vi "Impedance.vi"(7 "Auto Range (F: Off)":bool, 8 "error in (no error)":errorcluster, 9 "Imp Range (Ohm) (0.0)":dbl min=0.0 max=100000000.0 step=1.0 format="%.4f", 10 "Imp Type (0: CPD)":u32(ring) items=["CPD", "CPQ", "CPG", "CPRP", "CSD", "CSQ", "CSRS", "LPQ", "LPD", "LPG", "LPRP", "LSD", "LSQ", "LSRS", "RX", "ZTD", "ZTR", "GB", "YTD", "YTR"], 11 "VISA resource name":refnum<visa-resource-name>) -> (0 "error out":errorcluster, 3 "VISA resource name out":refnum<visa-resource-name>)   [LabVIEW 2015, in "Agilent 428X Series.lvlib"]
doc: "This control sets the measurement range and impedance type. Any value can be used as the setting value. The HP 428XA selects an appropriate measurement range for the setting value.\n\nWarning:\n\nIf this command is received while auto range is ON, the auto range function automatically set to OFF and the range will be held at the range dictated by the received command."
uses:
  Agilent 428X Series.lvlib
panel:
  # "On\nOff"
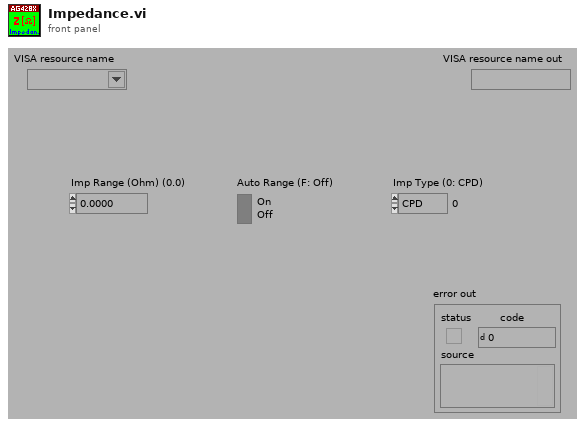
[diagram p1: front panel]
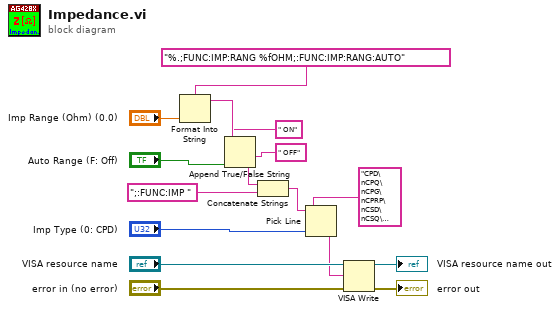
[diagram p0: block diagram]
diagram:
  n1 = Format Into String(format string="%.;FUNC:IMP:RANG %fOHM;:FUNC:IMP:RANG:AUTO", "Imp Range (Ohm) (0.0)") -> (resulting string=w10:string)  [unwired: 2 in, 1 out]
  n2 = Append True/False String(1:"Auto Range (F: Off)", 2:" OFF", 3:" ON", 4:w10) -> (0:w5:string)
  n3 = Concatenate Strings(w5, ";:FUNC:IMP ") -> (w4:string)
  n4 = Pick Line(string ("")=w4, multi-line string="CPD\nCPQ\nCPG\nCPRP\nCSD\nCSQ\nCSRS\nLPQ\nLPD\nLPG\nLPRP\nLSD\nLSQ\nLSRS\nRX\nZTD\nZTR\nGB\nYTD\nYTR", line index="Imp Type (0: CPD)") -> (output string=w1:string)
  n5 = VISA Write(VISA resource name="VISA resource name", write buffer=w1, error in (no error)="error in (no error)") -> (VISA resource name out=→"VISA resource name out":refnum<visa-resource-name>, error out=→"error out":errorcluster)  [unwired: 1 out]
